vi "Command_Joint_Angles_msg.vi"(5 "node":string, 6 "error in":errorcluster, 7 "JointCommand In":T1={"Mode"=enum."Position", "Arm Angles"=[], "Angle Names"=["_s0", "_s1", "_e0", "_e1", "_w0", "_w1", "_w2"]}) -> (0 "error out":errorcluster, 3 "JointCommand":T1={"Mode"=enum."Position", "Arm Angles"=[], "Angle Names"=["_s0", "_s1", "_e0", "_e1", "_w0", "_w1", "_w2"]})   [LabVIEW 2013]
uses:
  ROS/RosMessages/Clusters/JointCommand.ctl
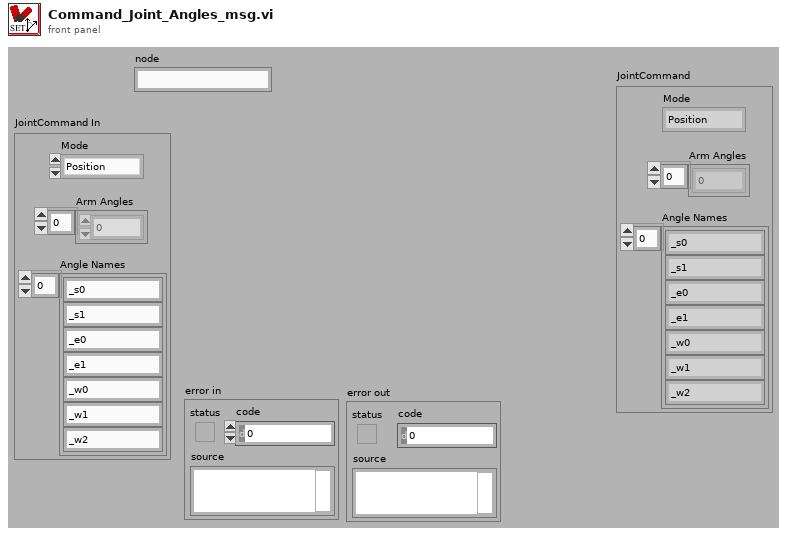
[diagram p1: front panel]
types:
  T1 = typedef "JointCommand.ctl" = cluster{"Mode":enum32{"", "Position", "Velocity", "Effort"}, "Arm Angles":dbl[], "Angle Names":string[]}
  T2 = typedef "_ROSControl.ctl" = cluster{"topic port":u16, "Node":string, "topic":string, "type":string, "node port":u32, "error ":errorcluster, "Direction":T3, "APIs":string[]}
  T3 = typedef "_ROSDirection.ctl" = enum16{"Node", "Publisher", "Subscriber", "Service Client"}
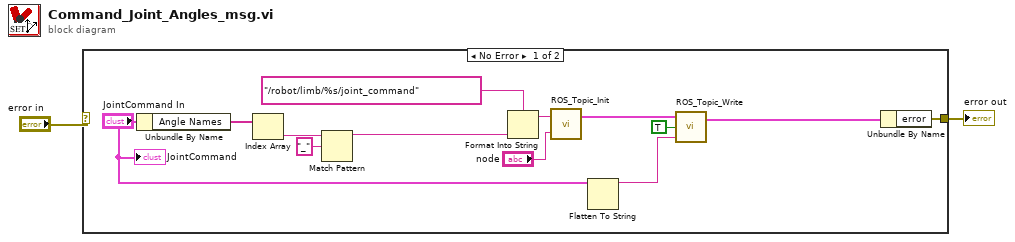
[diagram p0: block diagram]
diagram:
  n1 = case shown="No Error" "error in" {
    selector: "error in" -> [_ w16]
    tunnel: [w15 w16] -> w2
    frame No Error {
      n2 = Unbundle By Name("JointCommand In") -> ("Angle Names"=w4:string[])
      n3 = Index Array(array=w4) -> (element=w7:string)  [unwired: 1 in]
      n4 = Match Pattern(string=w7, regular expression="_") -> (before substring=w5:string)  [unwired: 1 in, 3 out]
      n5 = Format Into String(format string="/robot/limb/%s/joint_command" ("topic"), w5) -> (resulting string=w13:string)  [unwired: 2 in, 1 out]
      n6 = call "ROS_Topic_Init.vi"("node"="node", "topic"=w13) -> ("ROS out"=w12:T2)  [unwired: 1 in]
      n7 = Flatten To String(anything="JointCommand In") -> (data string=w8:string)  [unwired: 3 in, 2 out]
      n8 = call "ROS_Topic_Write.vi"("Msg in"=w8, "Continuous?"=TRUE, "ROS in"=w12) -> ("ROS out"=w11:T2)  [unwired: 1 in]
      n9 = Unbundle By Name(w11) -> ("error"=w15:errorcluster)
      "JointCommand" <- "JointCommand In"
    }
    frame Error {
    }
  }
  "error out" <- w2
